vi "Untitled 1 (1).vi"() -> ()   [LabVIEW 2020]
panel:
  out "agotado 3":string="Articulo agotado"
  in  "# dulce":dbl
  in  "#bebida fria":dbl
  in  "#cafe":dbl
  in  "# snack":dbl
  in  "stop":bool
  in  "Tab Control":enum32{"Page 1", "Page 2"}(tab)
  out "producto":bool
  out "cambio":bool
  in  "dulce":bool
  in  "bebida fria":bool
  in  "cafe":bool
  in  "snack":bool
  in  "Cancelar":bool
  in  "comprar":bool
  in  "Monedas":cluster{"moneda 10":bool, "moneda 20":bool}
  out "Cambio":dbl
  out "Dinero ingresado":dbl
  out "agotado":string="Articulo agotado"
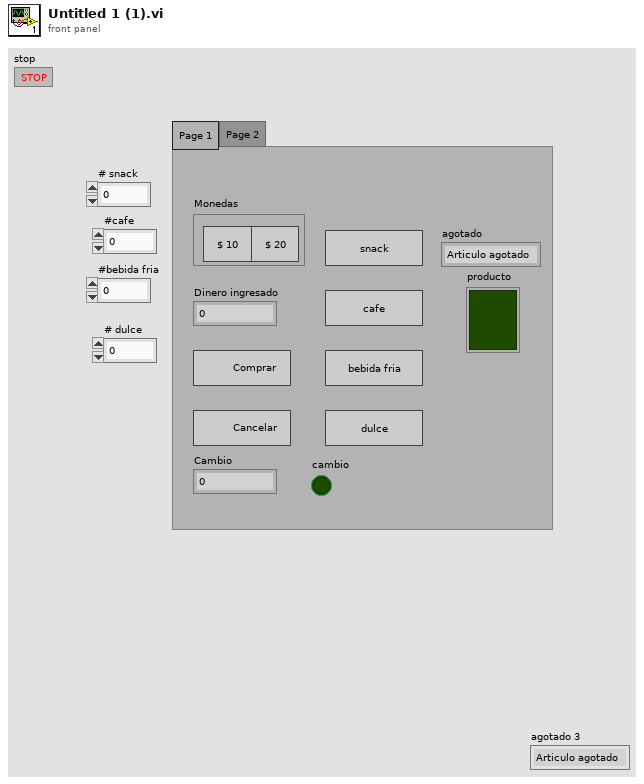
[diagram p1: front panel]
types:
  T1 = enum16{"inicio", "snack", "comprar s", "cambio s", "cafe", "comprar c", "cambio c", "bebida fria", "comprar bf", "cambio bf", "dulce", "comprar d", "cambio d", "reinicio", "cancelar"}
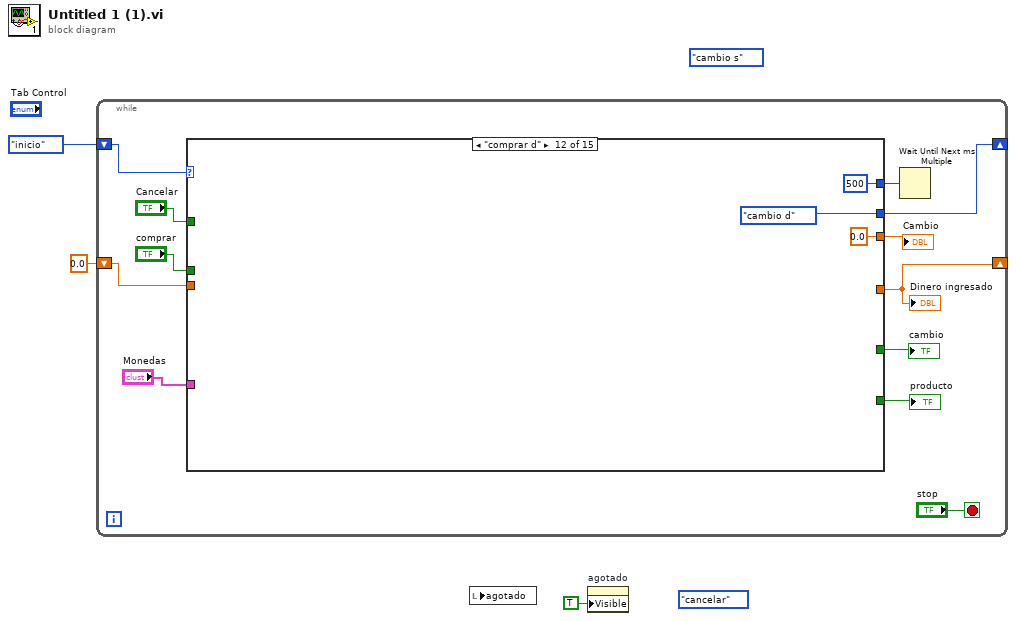
[diagram p0: block diagram]
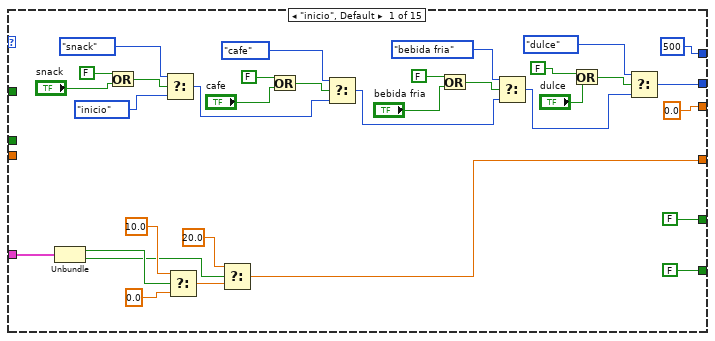
[diagram p2: hidden frame]
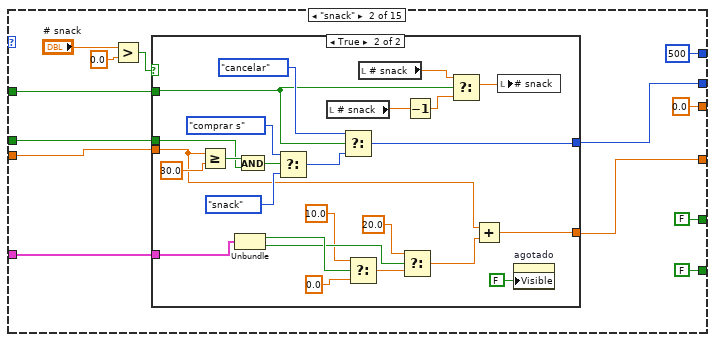
[diagram p3: hidden frame]
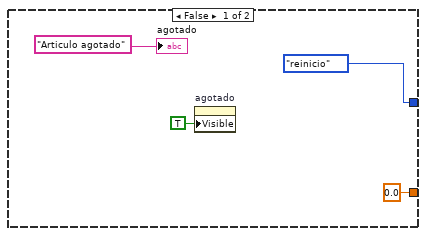
[diagram p4: hidden frame]
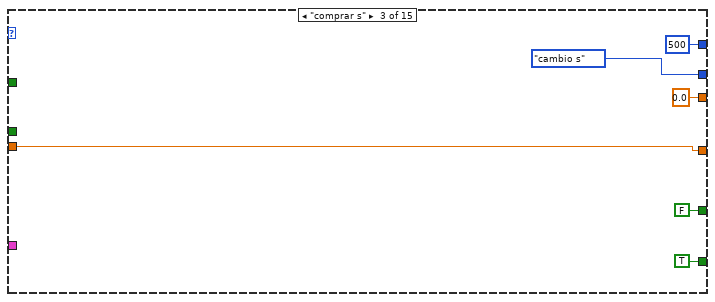
[diagram p5: hidden frame]
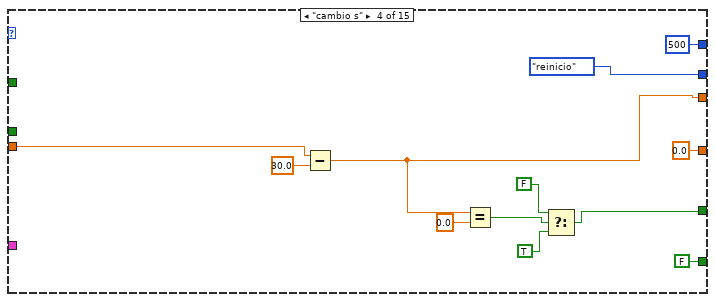
[diagram p6: hidden frame]
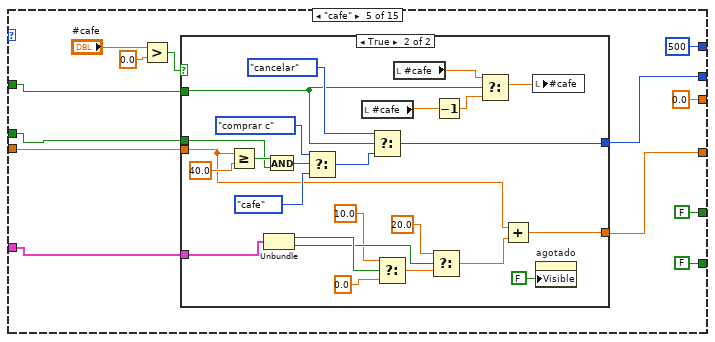
[diagram p7: hidden frame]
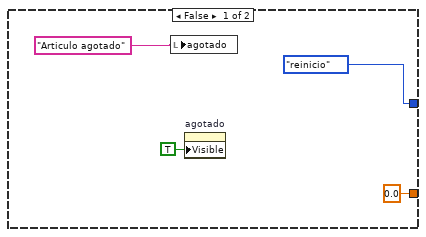
[diagram p8: hidden frame]
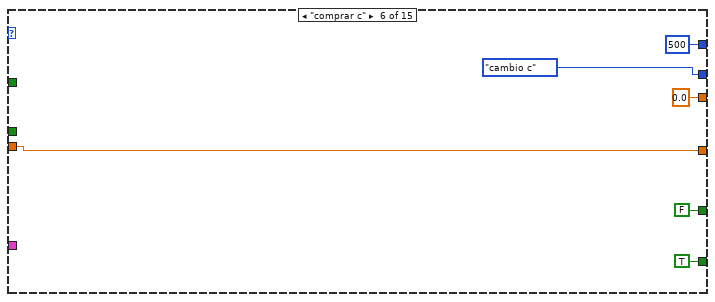
[diagram p9: hidden frame]
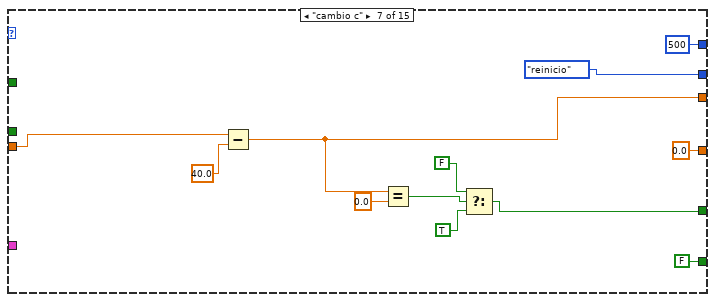
[diagram p10: hidden frame]
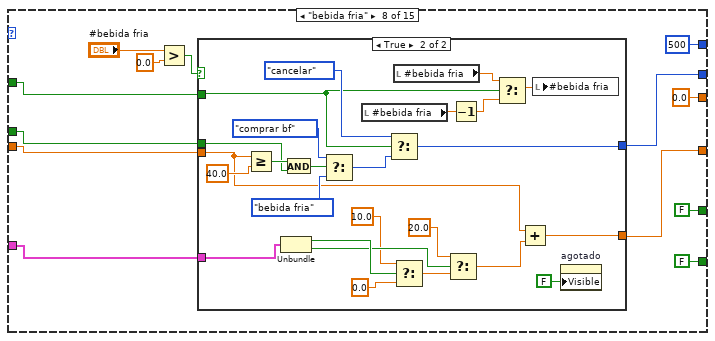
[diagram p11: hidden frame]
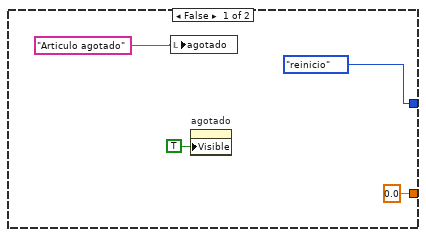
[diagram p12: hidden frame]
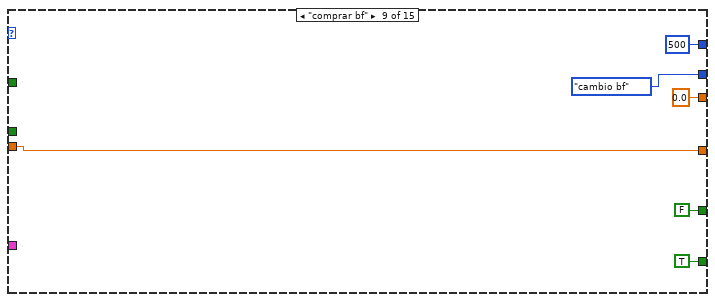
[diagram p13: hidden frame]
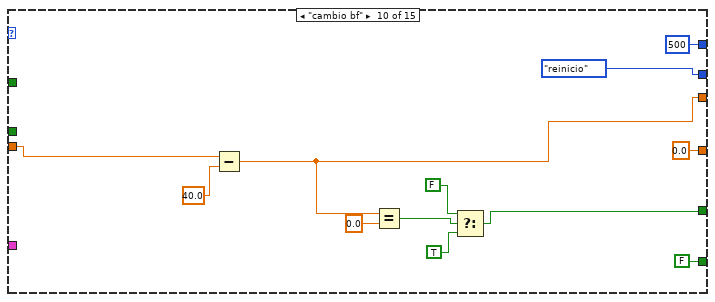
[diagram p14: hidden frame]
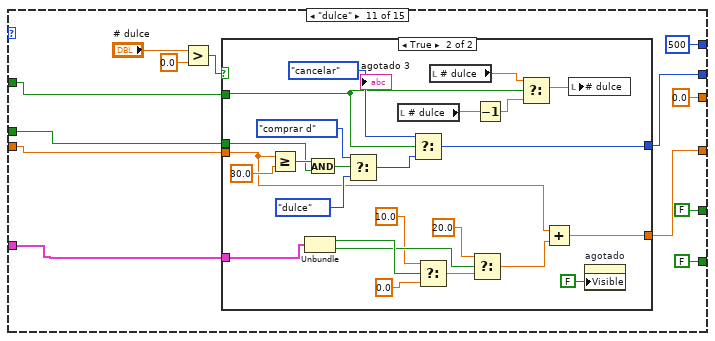
[diagram p15: hidden frame]
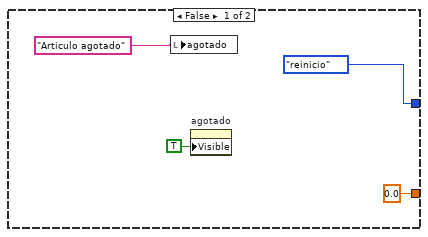
[diagram p16: hidden frame]
diagram:
  (unwired) T1."cancelar"
  (unwired) T1."cambio s"
  n1 = while {
    shift-right: [w13] -> _
    shift-left: T1."inicio" -> [w15]
    shift-right: [w7] -> _
    shift-left: 0.0 ("f") -> [w6]
    stop <- "stop" stop-if-true
    n2 = case shown="\"comprar d\"" w15 {
      tunnel: [500 500 500 500 500 500 500 500 500 500 500 500 _ _ _] -> w14
      tunnel: [w27 w53 T1."cambio s" T1."reinicio" w114 T1."cambio c" T1."reinicio" w174 T1."cambio bf" T1."reinicio" w233 T1."cambio d" _ _ _] -> w13
      tunnel: [0.0 0.0 0.0 w105 0.0 0.0 w159 0.0 0.0 w221 0.0 0.0 _ _ _] -> w12
      tunnel: "Monedas" -> [w25 w55 _ _ w115 _ _ w175 _ _ w238 _ _ _ _]
      tunnel: [w18 w54 w93 0.0 ("f") w113 w156 0.0 ("f") w171 w213 0.0 ("f") w232 _ _ _ _] -> w7
      tunnel: [FALSE FALSE TRUE FALSE FALSE TRUE FALSE FALSE TRUE FALSE FALSE _ _ _ _] -> w10
      tunnel: [FALSE FALSE FALSE w101 FALSE FALSE w161 FALSE FALSE w219 FALSE _ _ _ _] -> w9
      tunnel: w6 -> [_ w58 w93 w108 w116 w156 w157 w176 w213 w217 w237 _ _ _ _]
      tunnel: "comprar" -> [_ w57 _ _ w117 _ _ w177 _ _ w236 _ _ _ _]
      tunnel: "Cancelar" -> [_ w56 _ _ w118 _ _ w178 _ _ w235 _ _ _ _]
      frame "inicio", Default {
        n3 = Unbundle(w25) -> ("moneda 10"=w24:bool, "moneda 20"=w20:bool)
        n4 = Or(x=FALSE, y="snack") -> (x .or. y?=w46:bool)
        n5 = Select(t=T1."snack", s=w46, f=T1."inicio") -> (s? t:f=w39:T1)
        n6 = Select(t=10.0, s=w24, f=0.0) -> (s? t:f=w21:dbl)
        n7 = Select(t=20.0, s=w20, f=w21) -> (s? t:f=w18:dbl)
        n8 = Or(x=FALSE, y="cafe") -> (x .or. y?=w42:bool)
        n9 = Select(t=T1."cafe", s=w42, f=w39) -> (s? t:f=w34:T1)
        n10 = Or(x=FALSE, y="bebida fria") -> (x .or. y?=w37:bool)
        n11 = Select(t=T1."bebida fria", s=w37, f=w34) -> (s? t:f=w29:T1)
        n12 = Or(x=FALSE, y="dulce") -> (x .or. y?=w32:bool)
        n13 = Select(t=T1."dulce", s=w32, f=w29) -> (s? t:f=w27:T1)
      }
      frame "snack" {
        n14 = Greater?(x="# snack", y=0.0) -> (0:w59:bool)
        n15 = case shown="True" w59 {
          tunnel: w58 -> [_ w74]
          tunnel: w57 -> [_ w85]
          tunnel: w56 -> [_ w72]
          tunnel: w55 -> [_ w76]
          tunnel: [0.0 w73] -> w54
          tunnel: [T1."reinicio" w67] -> w53
          frame False {
            n16 = property on="agotado" class="Str"("Visible"=TRUE) -> ()  [unwired: 2 in, 2 out]
            "agotado" <- "Articulo agotado"
          }
          frame True {
            n17 = Greater Or Equal?(x=w74, y=30.0) -> (x >= y?=w89:bool)
            n18 = Unbundle(w76) -> ("moneda 10"=w82:bool, "moneda 20"=w80:bool)
            n19 = And(x=w89, y=w85) -> (x .and. y?=w90:bool)
            n20 = Select(t=T1."comprar s", s=w90, f=T1."snack") -> (s? t:f=w84:T1)
            n21 = local read "# snack"() -> (w71:dbl)
            n22 = Select(t=T1."cancelar", s=w72, f=w84) -> (s? t:f=w67:T1)
            n23 = Select(t=10.0, s=w82, f=0.0) -> (s? t:f=w81:dbl)
            n24 = local read "# snack"() -> (w68:dbl)
            n25 = Select(t=20.0, s=w80, f=w81) -> (s? t:f=w75:dbl)
            n26 = Decrement(x=w71) -> (x-1=w70:dbl)
            n27 = Select(t=w68, s=w72, f=w70) -> (s? t:f=w69:dbl)
            n28 = Add(x=w74, y=w75) -> (x+y=w73:dbl)
            n29 = local write "# snack"(w69) -> ()
            n30 = property on="agotado" class="Str"("Visible"=FALSE) -> ()  [unwired: 2 in, 2 out]
          }
        }
      }
      frame "comprar s" {
      }
      frame "cambio s" {
        n31 = Subtract(x=w108, y=30.0) -> (x-y=w105:dbl)
        n32 = Equal?(x=w105, y=0.0) -> (x = y?=w103:bool)
        n33 = Select(t=FALSE, s=w103, f=TRUE) -> (s? t:f=w101:bool)
      }
      frame "cafe" {
        n34 = Greater?(x="#cafe", y=0.0) -> (0:w119:bool)
        n35 = case shown="True" w119 {
          tunnel: w116 -> [_ w134]
          tunnel: w117 -> [_ w145]
          tunnel: w118 -> [_ w132]
          tunnel: w115 -> [_ w136]
          tunnel: [0.0 w133] -> w113
          tunnel: [T1."reinicio" w127] -> w114
          frame False {
            n36 = local write "agotado"("Articulo agotado") -> ()
            n37 = property on="agotado" class="Str"("Visible"=TRUE) -> ()  [unwired: 2 in, 2 out]
          }
          frame True {
            n38 = Greater Or Equal?(x=w134, y=40.0) -> (x >= y?=w149:bool)
            n39 = Unbundle(w136) -> ("moneda 10"=w142:bool, "moneda 20"=w140:bool)
            n40 = And(x=w149, y=w145) -> (x .and. y?=w150:bool)
            n41 = Select(t=T1."comprar c", s=w150, f=T1."cafe") -> (s? t:f=w144:T1)
            n42 = local read "#cafe"() -> (w131:dbl)
            n43 = Select(t=T1."cancelar", s=w132, f=w144) -> (s? t:f=w127:T1)
            n44 = Select(t=10.0, s=w142, f=0.0) -> (s? t:f=w141:dbl)
            n45 = local read "#cafe"() -> (w128:dbl)
            n46 = Select(t=20.0, s=w140, f=w141) -> (s? t:f=w135:dbl)
            n47 = Decrement(x=w131) -> (x-1=w130:dbl)
            n48 = Select(t=w128, s=w132, f=w130) -> (s? t:f=w129:dbl)
            n49 = Add(x=w134, y=w135) -> (x+y=w133:dbl)
            n50 = local write "#cafe"(w129) -> ()
            n51 = property on="agotado" class="Str"("Visible"=FALSE) -> ()  [unwired: 2 in, 2 out]
          }
        }
      }
      frame "comprar c" {
      }
      frame "cambio c" {
        n52 = Subtract(x=w157, y=40.0) -> (x-y=w159:dbl)
        n53 = Equal?(x=w159, y=0.0) -> (x = y?=w164:bool)
        n54 = Select(t=FALSE, s=w164, f=TRUE) -> (s? t:f=w161:bool)
      }
      frame "bebida fria" {
        n55 = Greater?(x="#bebida fria", y=0.0) -> (0:w179:bool)
        n56 = case shown="True" w179 {
          tunnel: w176 -> [_ w194]
          tunnel: w177 -> [_ w205]
          tunnel: w178 -> [_ w192]
          tunnel: w175 -> [_ w196]
          tunnel: [0.0 w193] -> w171
          tunnel: [T1."reinicio" w187] -> w174
          frame False {
            n57 = local write "agotado"("Articulo agotado") -> ()
            n58 = property on="agotado" class="Str"("Visible"=TRUE) -> ()  [unwired: 2 in, 2 out]
          }
          frame True {
            n59 = Greater Or Equal?(x=w194, y=40.0) -> (x >= y?=w209:bool)
            n60 = Unbundle(w196) -> ("moneda 10"=w202:bool, "moneda 20"=w200:bool)
            n61 = And(x=w209, y=w205) -> (x .and. y?=w210:bool)
            n62 = Select(t=T1."comprar bf", s=w210, f=T1."bebida fria") -> (s? t:f=w204:T1)
            n63 = local read "#bebida fria"() -> (w191:dbl)
            n64 = Select(t=T1."cancelar", s=w192, f=w204) -> (s? t:f=w187:T1)
            n65 = local read "#bebida fria"() -> (w188:dbl)
            n66 = Select(t=10.0, s=w202, f=0.0) -> (s? t:f=w201:dbl)
            n67 = Select(t=20.0, s=w200, f=w201) -> (s? t:f=w195:dbl)
            n68 = Decrement(x=w191) -> (x-1=w190:dbl)
            n69 = Select(t=w188, s=w192, f=w190) -> (s? t:f=w189:dbl)
            n70 = Add(x=w194, y=w195) -> (x+y=w193:dbl)
            n71 = local write "#bebida fria"(w189) -> ()
            n72 = property on="agotado" class="Str"("Visible"=FALSE) -> ()  [unwired: 2 in, 2 out]
          }
        }
      }
      frame "comprar bf" {
      }
      frame "cambio bf" {
        n73 = Subtract(x=w217, y=40.0) -> (x-y=w221:dbl)
        n74 = Equal?(x=w221, y=0.0) -> (x = y?=w224:bool)
        n75 = Select(t=FALSE, s=w224, f=TRUE) -> (s? t:f=w219:bool)
      }
      frame "dulce" {
        n76 = Greater?(x="# dulce", y=0.0) -> (0:w240:bool)
        n77 = case shown="True" w240 {
          tunnel: w237 -> [_ w254]
          tunnel: w236 -> [_ w265]
          tunnel: w235 -> [_ w252]
          tunnel: w238 -> [_ w256]
          tunnel: [0.0 w253] -> w232
          tunnel: [T1."reinicio" w247] -> w233
          frame False {
            n78 = local write "agotado"("Articulo agotado") -> ()
            n79 = property on="agotado" class="Str"("Visible"=TRUE) -> ()  [unwired: 2 in, 2 out]
          }
          frame True {
            n80 = Greater Or Equal?(x=w254, y=30.0) -> (x >= y?=w269:bool)
            n81 = Unbundle(w256) -> ("moneda 10"=w262:bool, "moneda 20"=w260:bool)
            n82 = And(x=w269, y=w265) -> (x .and. y?=w270:bool)
            n83 = Select(t=T1."comprar d", s=w270, f=T1."dulce") -> (s? t:f=w264:T1)
            n84 = local read "# dulce"() -> (w251:dbl)
            n85 = Select(t=T1."cancelar", s=w252, f=w264) -> (s? t:f=w247:T1)
            n86 = Select(t=10.0, s=w262, f=0.0) -> (s? t:f=w261:dbl)
            n87 = local read "# dulce"() -> (w248:dbl)
            n88 = Select(t=20.0, s=w260, f=w261) -> (s? t:f=w255:dbl)
            n89 = Decrement(x=w251) -> (x-1=w250:dbl)
            n90 = Select(t=w248, s=w252, f=w250) -> (s? t:f=w249:dbl)
            n91 = Add(x=w254, y=w255) -> (x+y=w253:dbl)
            n92 = local write "# dulce"(w249) -> ()
            n93 = property on="agotado" class="Str"("Visible"=FALSE) -> ()  [unwired: 2 in, 2 out]
          }
        }
      }
      frame "comprar d" {
      }
      frame "cambio d" {
      }
      frame "reinicio" {
      }
      frame "cancelar" {
      }
    }
    "Cambio" <- w12
    "Dinero ingresado" <- w7
    "cambio" <- w9
    "producto" <- w10
    n94 = Wait Until Next ms Multiple(millisecond multiple=w14) -> ()  [unwired: 1 out]
  }
  n95 = local read "agotado"() -> ()  [unwired: 1 in]
  n96 = property on="agotado" class="Str"("Visible"=TRUE) -> ()  [unwired: 2 in, 2 out]
